vi "MW_Freq_Read.vi"(8 "错误输入（无错误）":errorcluster, 11 "VISA引用句柄输入":refnum<visa-resource-name>) -> (0 "错误输出":errorcluster, 2 "Freq(GHz)":dbl, 3 "VISA引用句柄输出":refnum<visa-resource-name>, 5 "read buffer":string)   [LabVIEW 2016, in "Microwave Source.lvlib"]
doc: "设置微波源输出功率。"
uses:
  Microwave Source.lvlib
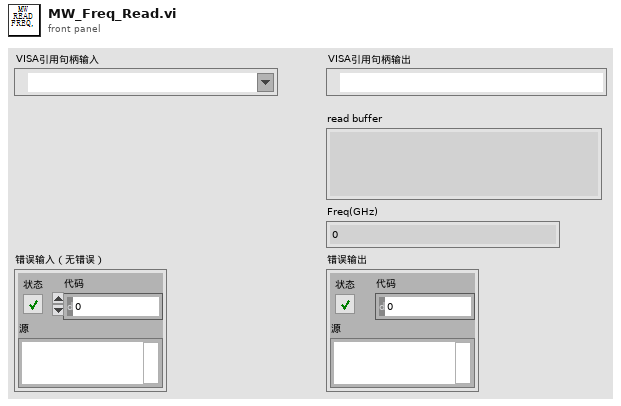
[diagram p1: front panel]
types:
  T1 = typedef "Microwave Source.lvlib/MW_ctl_DeviceType.ctl" = enum16{"R&S", "Other"}
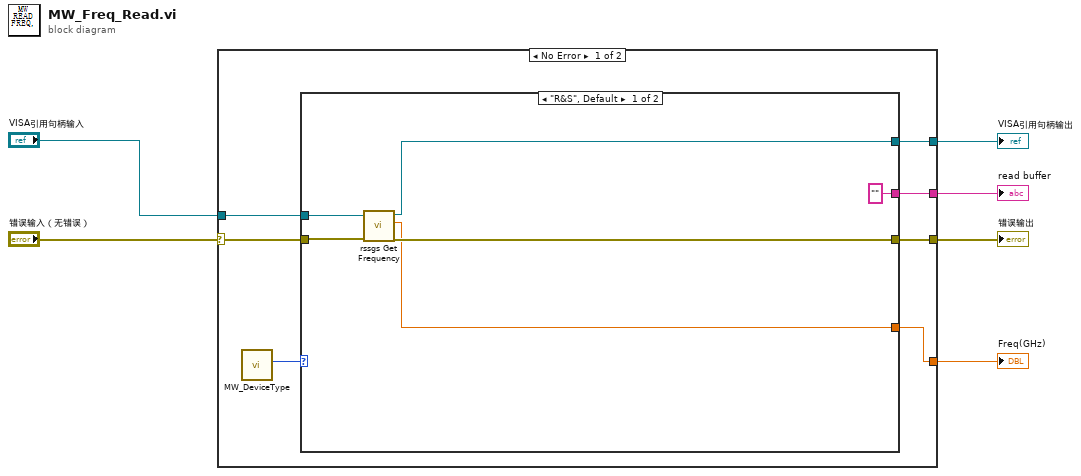
[diagram p0: block diagram]
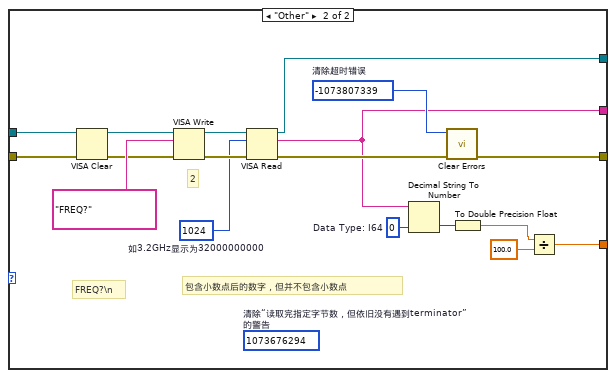
[diagram p2: hidden frame]
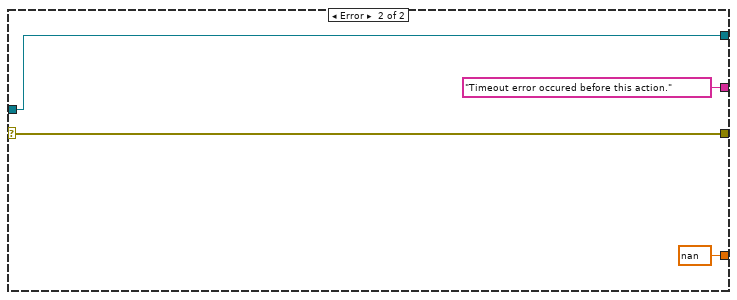
[diagram p3: hidden frame]
diagram:
  n1 = case shown="No Error" "错误输入（无错误）" {
    selector: "错误输入（无错误）" -> [w10 w41]
    tunnel: "VISA引用句柄输入" -> [w9 w40]
    tunnel: [w13 w40] -> w5
    tunnel: [w12 w41] -> w4
    tunnel: [w11 "Timeout error occured before this action." ("read buffer")] -> w3
    tunnel: [w8 nan] -> w2
    frame No Error {
      n2 = call "MW_DeviceType.vi"() -> ("DeviceType"=w7:T1)  [unwired: 11 in]
      n3 = case shown="\"R&S\", Default" w7 {
        tunnel: [w17 w36] -> w13
        tunnel: [w15 w30] -> w12
        tunnel: ["" ("read buffer") w29] -> w11
        tunnel: w10 -> [w19 w25]
        tunnel: w9 -> [w18 w23]
        tunnel: [w14 w20] -> w8
        frame "R&S", Default {
          n4 = call <instrlib>:"rssgs Get Frequency.vi"("error in (no error)"=w19, "VISA resource name"=w18) -> ("error out"=w15:errorcluster, "Frequency"=w14:dbl, "VISA resource name out"=w17:refnum<visa-resource-name>)  [unwired: 7 in]
        }
        frame "Other" {
          (unwired) 1073676294  # 清除“读取完指定字节数，但依旧没有遇到terminator”的警告
          w28 = i64 0  # Data Type: I64
          w32 = -1073807339  # 清除超时错误
          w33 = u32 1024  # 如3.2GHz显示为32000000000
          # "包含小数点后的数字，但并不包含小数点"
          # "FREQ?\\n"
          # "2"
          n5 = VISA Clear(VISA resource name=w23, error in (no error)=w25) -> (VISA resource name out=w22:refnum<visa-resource-name>, error out=w24:errorcluster)
          n6 = VISA Write(VISA resource name=w22, write buffer="FREQ?", error in (no error)=w24) -> (VISA resource name out=w37:refnum<visa-resource-name>, error out=w35:errorcluster)  [unwired: 1 out]
          n7 = VISA Read(VISA resource name=w37, byte count=w33, error in (no error)=w35) -> (VISA resource name out=w36:refnum<visa-resource-name>, read buffer=w29:string, error out=w31:errorcluster)  [unwired: 1 out]
          n8 = Decimal String To Number(string=w29, default (0L)=w28) -> (number=w27:i64)  [unwired: 1 in, 1 out]
          n9 = call <vilib>:"Clear Errors.vi"("error in (no error)"=w31, "specific error code to clear (0: all)"=w32) -> ("error out"=w30:errorcluster)  [unwired: 4 in, 1 out]
          n10 = To Double Precision Float(number=w27) -> (double precision float=w21:dbl)
          n11 = Divide(x=w21, y=100.0) -> (x/y=w20:dbl)
        }
      }
    }
    frame Error {
    }
  }
  "VISA引用句柄输出" <- w5
  "错误输出" <- w4
  "read buffer" <- w3
  "Freq(GHz)" <- w2
